vi "writeU64FIFO.vi"(8 "error in (no error)":errorcluster, 9 "Timeout":i32, 10 "Data":u64[](array[numeric]), 11 "TimestampControlFIFO in":refnum<class "TimestampControlFIFO.lvclass">) -> (0 "error out":errorcluster, 2 "ElementsRemaining":u32, 3 "TimestampControlFIFO out":refnum<class "TimestampControlFIFO.lvclass">)   [LabVIEW 2016, in "TimestampControlFIFO.lvclass"]
uses:
  TimestampControlFIFO.lvclass
  TimestampControlFIFO.lvclass/TimestampControlFIFO.ctl
  FPGA/FPGA.lvclass
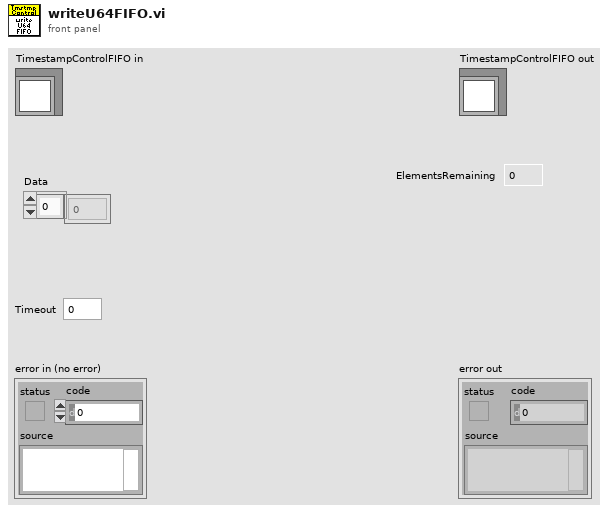
[diagram p1: front panel]
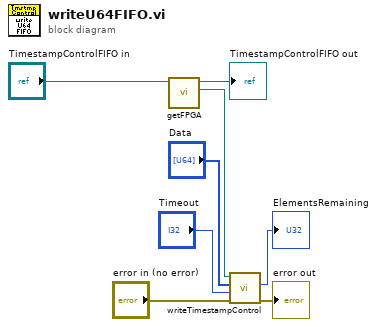
[diagram p0: block diagram]
diagram:
  n1 = call "getFPGA.vi"("TimestampControlFIFO in"="TimestampControlFIFO in") -> ("FPGA"=w6:refnum<class "FPGA.lvclass">, "TimestampControlFIFO out"=→"TimestampControlFIFO out":refnum<class "TimestampControlFIFO.lvclass">)  [unwired: 9 in]
  n2 = call "writeTimestampControl.vi"("error in (no error)"="error in (no error)", "Timeout"="Timeout", "Data"="Data", "FPGA in"=w6) -> ("error out"=→"error out":errorcluster, "ElementsRemaining"=→"ElementsRemaining":u32)  [unwired: 5 in, 1 out]
